vi "Main gScript UI.vi"() -> ()   [LabVIEW 2017]
uses:
  UI typedefs/gScript Controller Status.ctl
  gScript Interpreter/Type Definitions/Main Memory.ctl
  gScript Interpreter/Type Definitions/Memory Cell.ctl
  gScript Interpreter/Type Definitions/Memory Cell Type Enum.ctl
  gScript Interpreter/Type Definitions/Variable Table.ctl
  gScript Interpreter/Type Definitions/Variable.ctl
  Shared Components/Gantry Class/Type Definitions/Virtual Modes.ctl
  UI typedefs/gScript Controller Commands.ctl
  Shared Components/Gantry Class/Type Definitions/Init_Modes.ctl
  gScript Interpreter/gScript Interpreter.lvclass
  Application Utilities/Console Log/Console Log.lvclass
  Shared Components/Gantry Class/Gantry Class.lvclass
panel:
  out "Abort Async Request":bool=TRUE
  in  "Tab Control":enum32{"Control", "Memory"}(tab)
  in  "Execute":bool
  in  "Command Input":string
  in  "Virtual Mode":T1=enum."Virtual"
  out "Status":T2
  in  "Abort Script":bool
  in  "EXIT":bool
  in  "Config Root Directory":path
  in  "Pause Script":bool
  in  "Run Script":bool
  in  "Load Script":bool
  in  "Script Input":string
  in  "Save Script":bool
  out "Console":string
  in  "Variable Table":T3
  in  "Main Memory":T7
  in  "Memory Size":i32=16
  # "Documentation\nhttps://bit.ly/345jp8M"
  # "Command Input >"
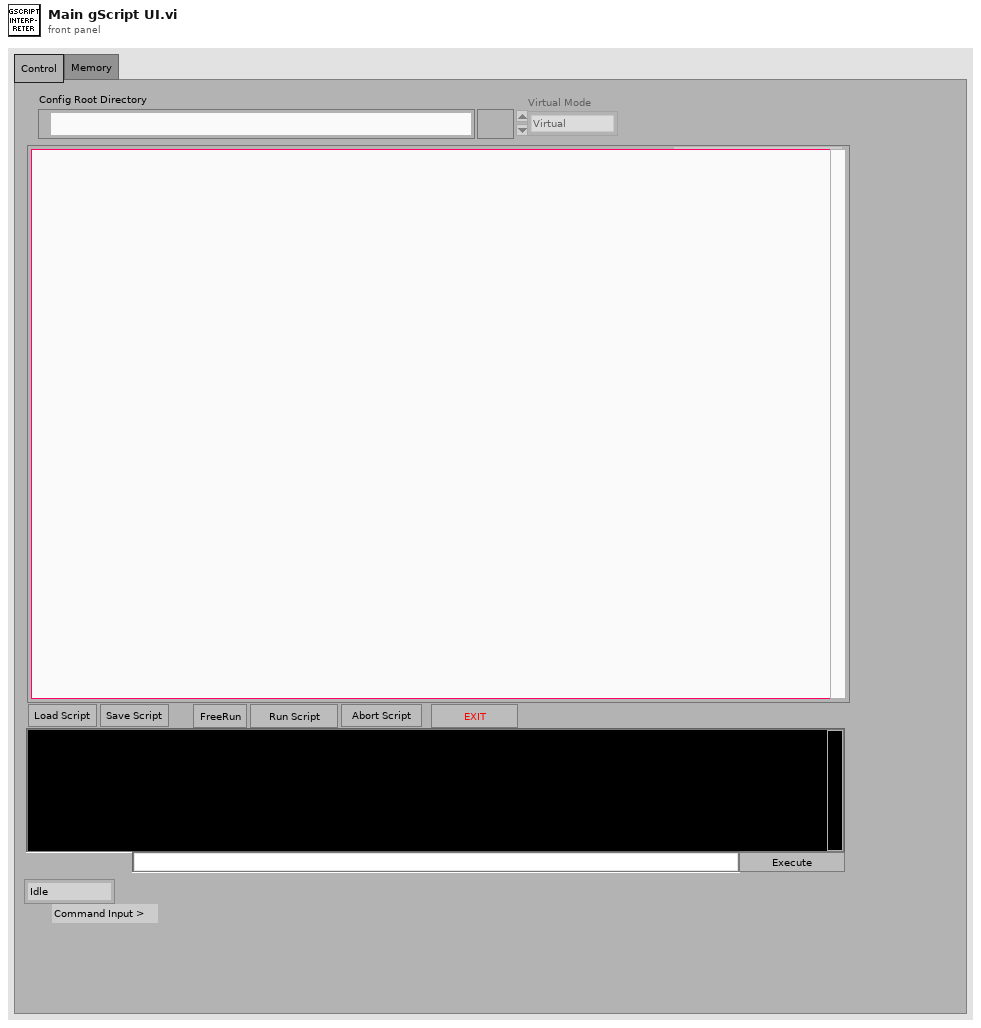
[diagram p1: front panel]
types:
  T1 = typedef "Virtual Modes.ctl" = enum16{"Nonvirtual", "Pseudovirtual", "Virtual"}
  T2 = typedef "gScript Controller Status.ctl" = enum16{"Idle", "Running", "Paused"}
  T3 = typedef "Variable Table.ctl" = T4[]
  T4 = typedef "Variable.ctl" = cluster{"Variable Name":string, "Memory Cell":T5}
  T5 = typedef "Memory Cell.ctl" = cluster{"type":T6, "x":dbl, "y":dbl, "z":dbl, "w":dbl}
  T6 = typedef "Memory Cell Type Enum.ctl" = enum16{"integer", "float", "vector", "rotation"}
  T7 = typedef "Main Memory.ctl" = T5[]
  T8 = enum8{"Enabled", "Disabled", "Disabled and Grayed Out"}
  T9 = typedef "gScript Controller Commands.ctl" = enum16{"Initialize", "Run Script", "Abort Script", "Exit", "Load Script", "Save Script", "Run Command"}
  T10 = cluster{"Variable Name":string, "Memory Cell":T5}[]
  T11 = typedef "Init_Modes.ctl" = enum16{"Full", "Robot Only", "Dispenser Only", "Cameras Only", "Robot and Cameras", "Robot and Cameras and Dispenser", "Manifold Only"}
  T12 = enum16{"open", "replace", "create", "open or create", "replace or create", "replace or create with confirmation"}
  T13 = cluster{"Shift":bool, "Ctrl":bool, "Alt":bool, "Cmd":bool, "Opt":bool}
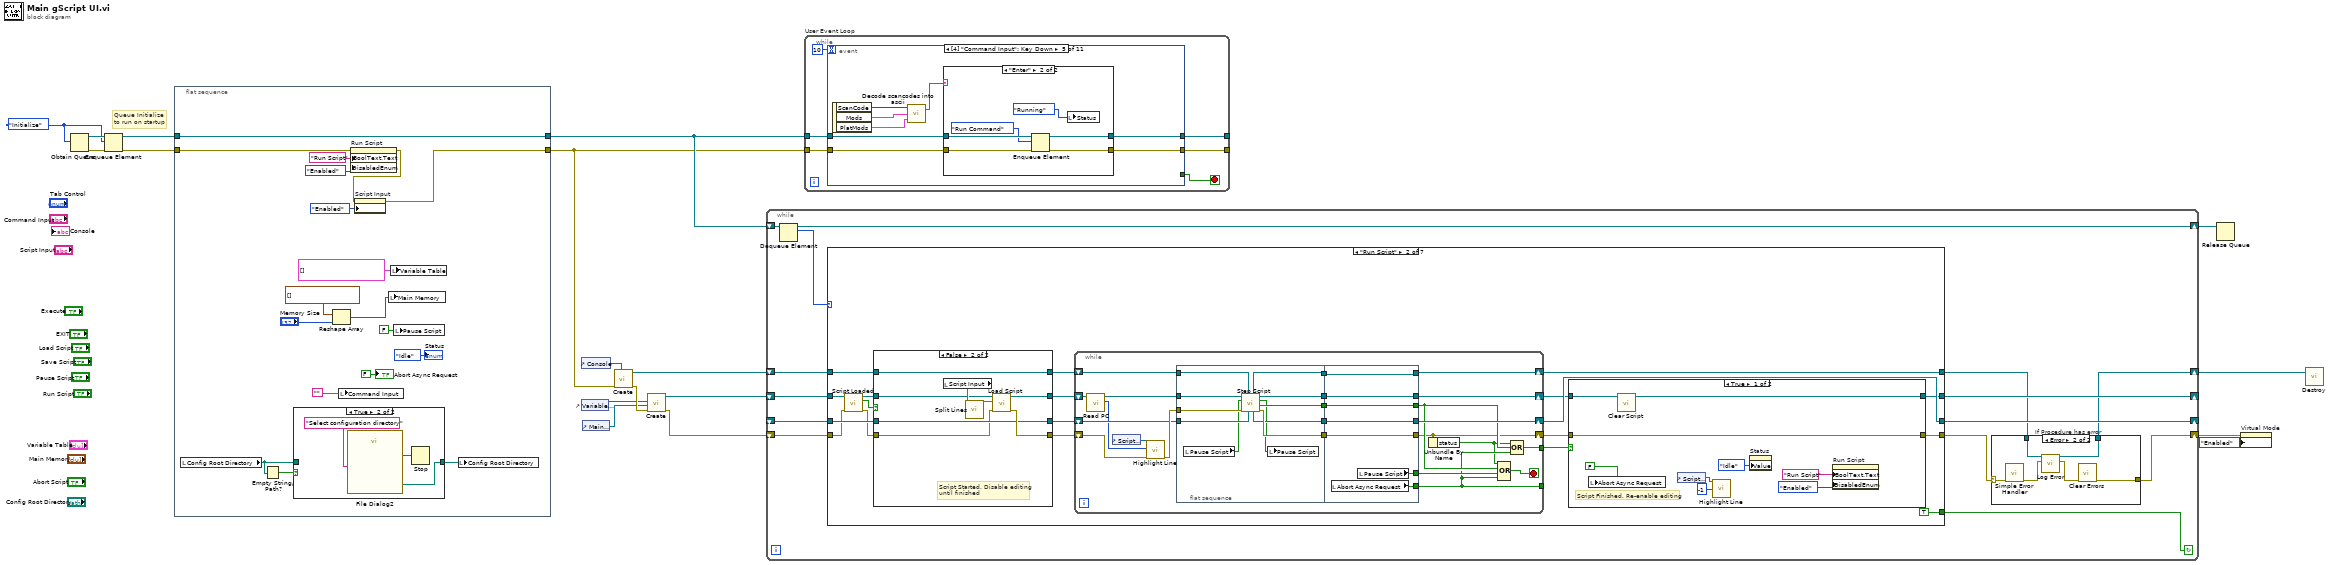
[diagram p0: block diagram]
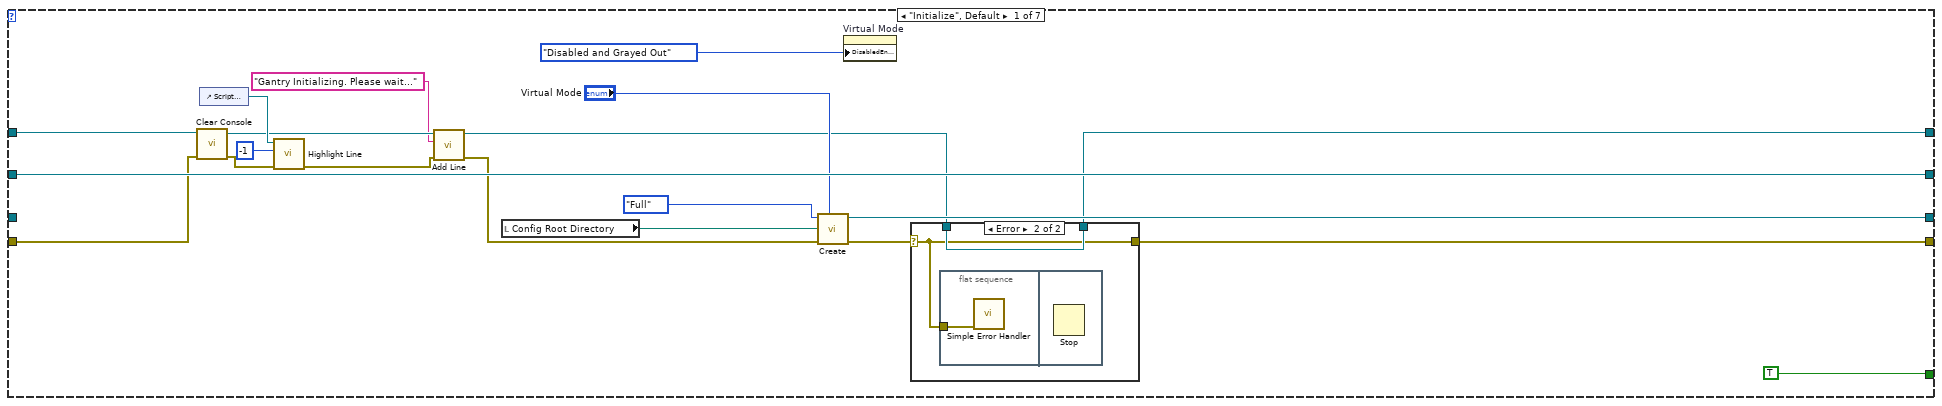
[diagram p4: hidden frame]
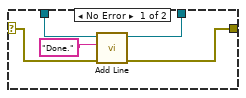
[diagram p5: hidden frame]
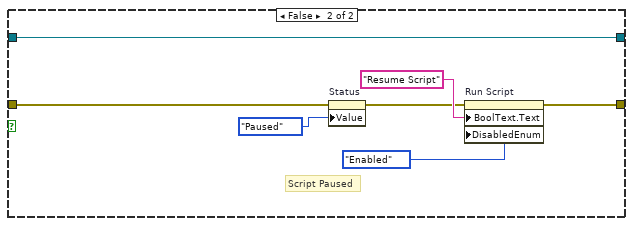
[diagram p7: hidden frame]
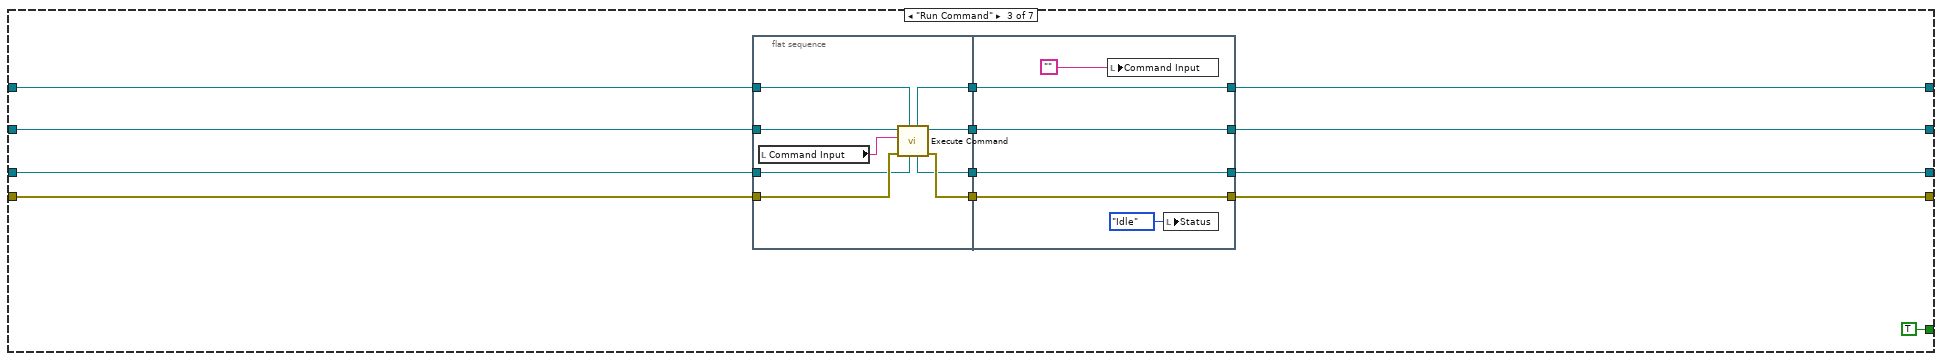
[diagram p8: hidden frame]
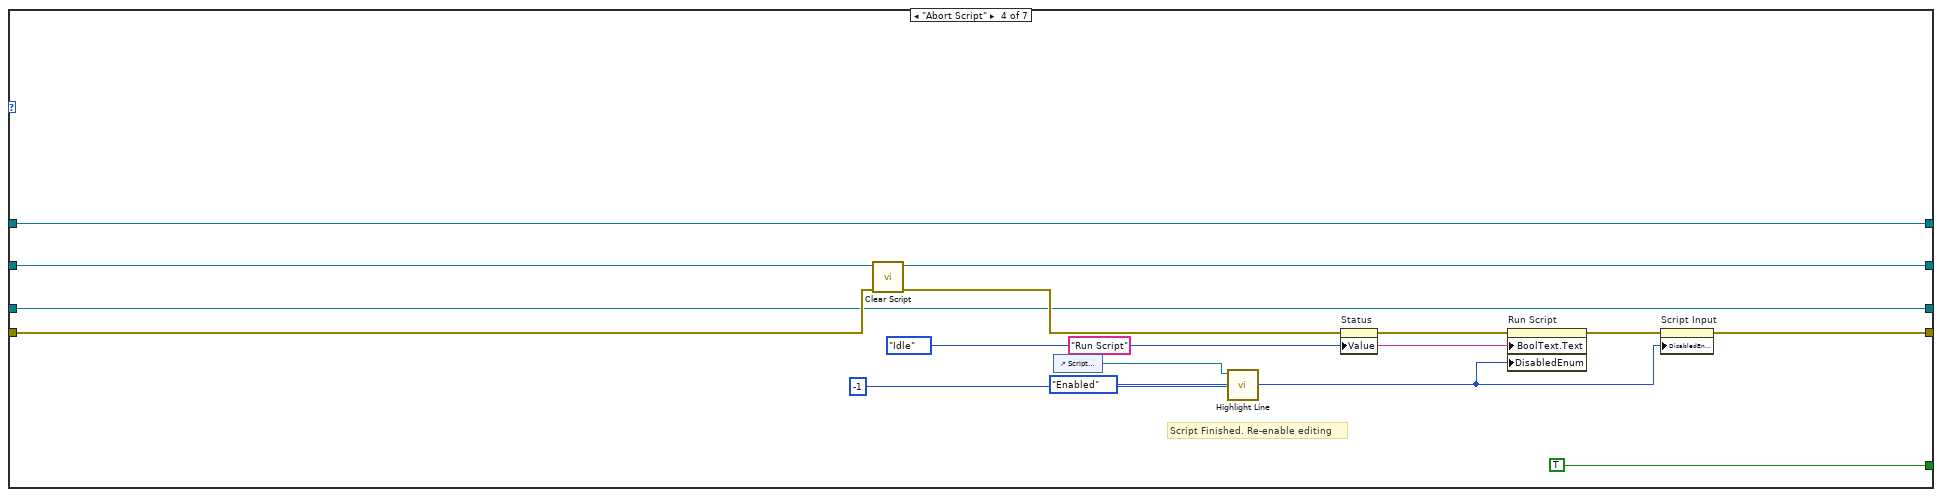
[diagram p9: hidden frame]
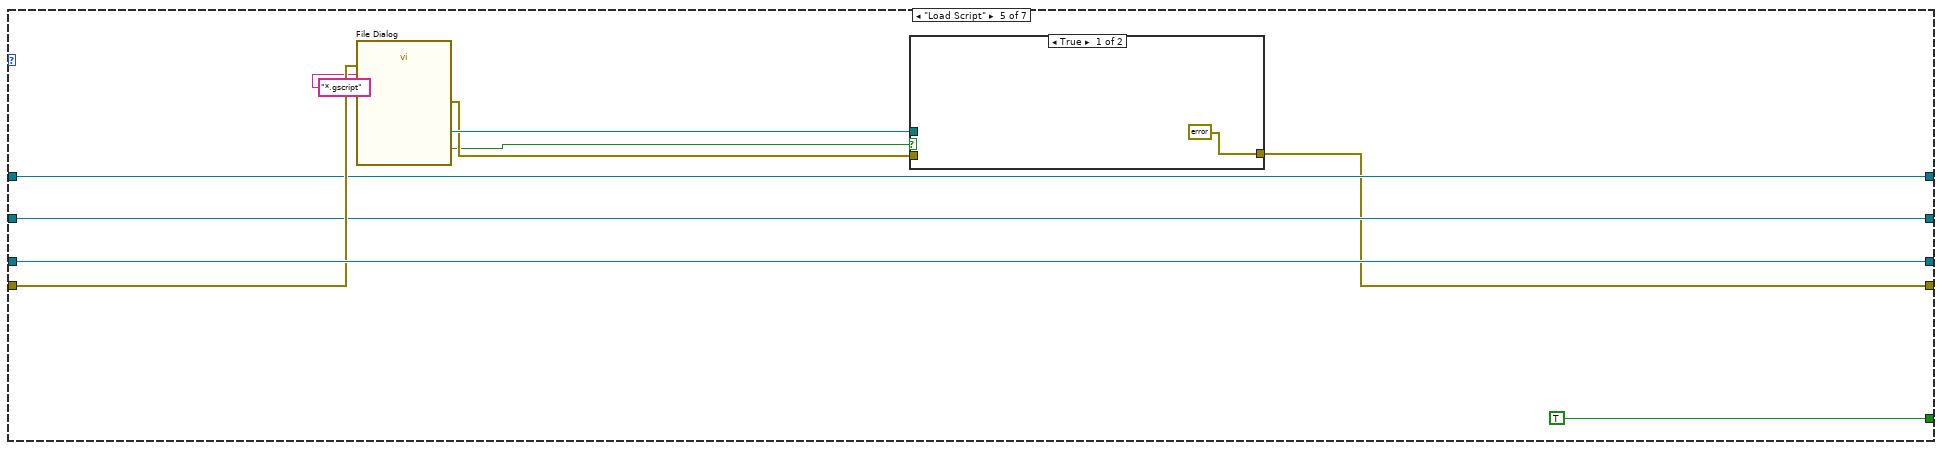
[diagram p10: hidden frame]
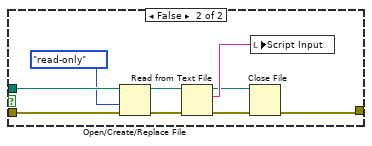
[diagram p11: hidden frame]
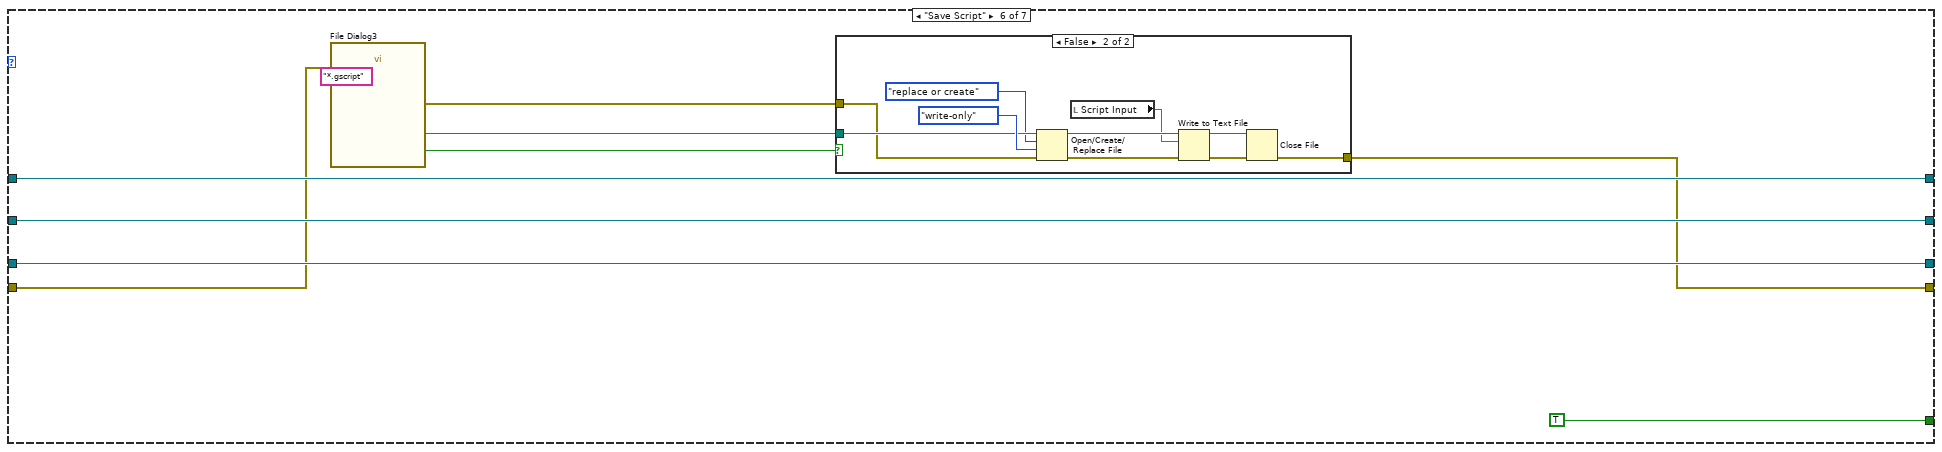
[diagram p12: hidden frame]
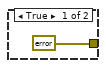
[diagram p13: hidden frame]
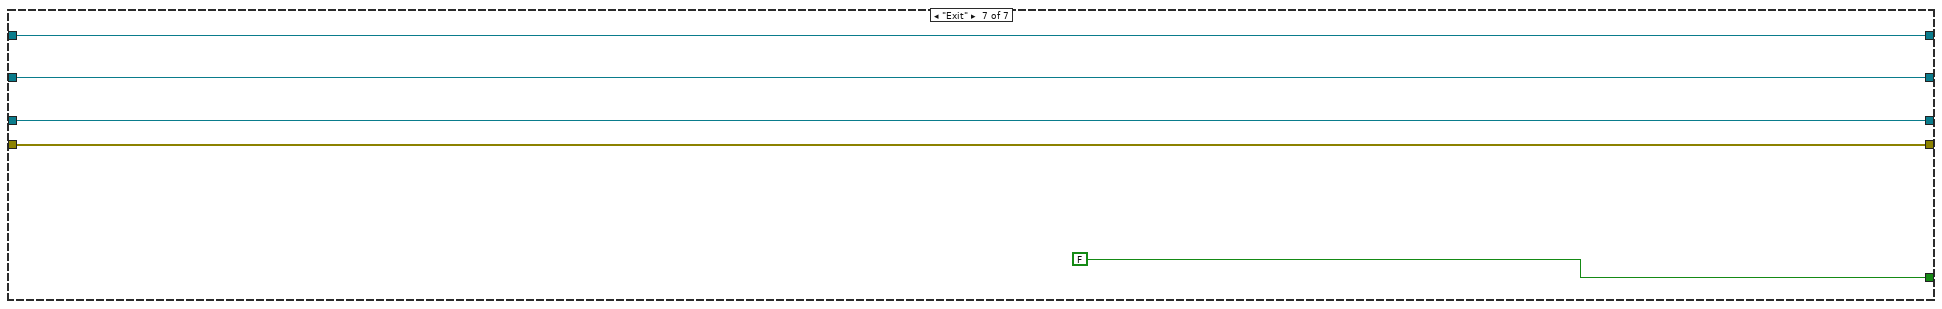
[diagram p14: hidden frame]
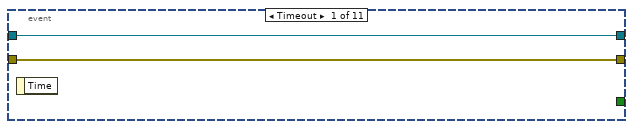
[diagram p15: hidden frame]
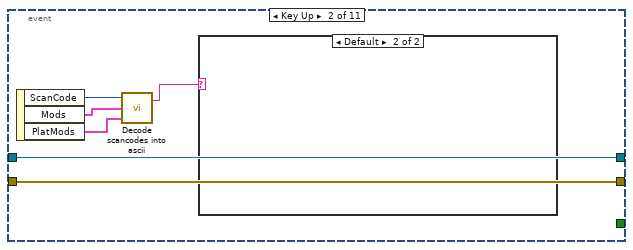
[diagram p16: hidden frame]
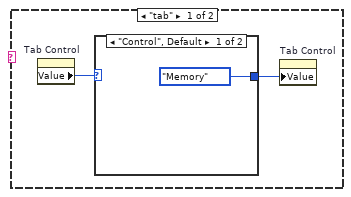
[diagram p17: hidden frame]
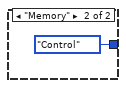
[diagram p18: hidden frame]
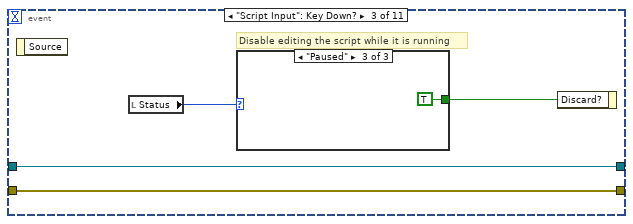
[diagram p19: hidden frame]
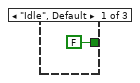
[diagram p20: hidden frame]
diagram:
  w15 = gScript_Controller_Commands."Initialize"
  # "Queue Initialize \nto run on startup"
  n1 = Obtain Queue(element data type=w15) -> (queue out=w17:refnum<queue>, error out=w16:errorcluster)  [unwired: 4 in, 1 out]
  n2 = Enqueue Element(queue=w17, element=w15, error in (no error)=w16) -> (queue out=w9:refnum<queue>, error out=w7:errorcluster)  [unwired: 1 in, 1 out]
  n3 = flat-sequence {
    tunnel: w9 -> [w36]
    tunnel: [w36] -> w8
    tunnel: w7 -> [w32]
    tunnel: [w29] -> w6
    frame #0 {
      n4 = local read "Config Root Directory"() -> (w22:path)
      n5 = Empty String/Path?(string/path=w22) -> (empty?=w21:bool)
      n6 = case shown="True" w21 {
        tunnel: w22 -> [w37 _]
        tunnel: [w37 w40] -> w20
        frame False {
        }
        frame True {
          n7 = call "File Dialog2"("prompt"="Select configuration directory") -> ("selected path"=w40:path, "cancelled"=w38:bool)  [unwired: 11 in, 2 out]
          n8 = Stop(stop? (T)=w38) -> ()
        }
      }
      n9 = Reshape Array(T5[] [] ("Main Memory"), "Memory Size") -> (w23:T5[])
      n10 = local write "Command Input"("") -> ()
      n11 = property on="Run Script" class="Bool (strict)"(error in=w32, "BoolText.Text"="Run Script" ("Boolean Text.Text"), "DisabledEnum"=T8."Enabled" ("Disabled")) -> (error out=w30:errorcluster)  [unwired: 1 in, 1 out]
      n12 = property on="Script Input" class="Str"(error in=w30, "DisabledEnum"=T8."Enabled" ("Disabled")) -> (error out=w29:errorcluster)  [unwired: 1 in, 1 out]
      n13 = local write "Main Memory"(w23) -> ()
      n14 = local write "Variable Table"(T10 [] ("Variable Table")) -> ()
      n15 = local write "Pause Script"(FALSE ("Pause Script")) -> ()
      n16 = local write "Config Root Directory"(w20) -> ()
      "Status" <- gScript_Controller_Status."Idle" ("Status")
      "Abort Async Request" <- FALSE ("Abort Requested")
    }
  }
  n17 = control-ref of="Variable Table"() -> (w4:refnum<vi>)
  n18 = control-ref of="Console"() -> (w18:refnum<vi>)
  n19 = control-ref of="Main Memory"() -> (w3:refnum<vi>)
  n20 = call "Create.vi"("Console"=w18, "error in"=w6) -> ("error out"=w11:errorcluster, "Console Log out"=w14:refnum<class "Console Log.lvclass">)  [unwired: 8 in]
  n21 = call "Create.vi"("error in (no error)"=w11, "Main Memory Ref"=w3, "Variable Table Ref"=w4) -> ("error out"=w10:errorcluster, "gScript Interpreter out"=w13:refnum<class "gScript Interpreter.lvclass">)  [unwired: 7 in]
  n22 = while {
    shift-right: [w41] -> w12
    shift-left: w14 -> [w52]
    shift-right: [w46] -> _
    shift-left: w13 -> [w51]
    shift-right: [w49] -> _
    shift-left: _ -> [w50]
    shift-right: [w43] -> w2
    shift-left: w10 -> [w48]
    shift-right: [w45] -> w5
    shift-left: w8 -> [w54]
    stop <- w47 continue-if-true
    n23 = Dequeue Element(queue=w54) -> (queue out=w45:refnum<queue>, element=w53:T9)  [unwired: 2 in, 2 out]
    n24 = case shown="\"Run Script\"" w53 {
      tunnel: w52 -> [w78 w100 w189 w211 w227 w249 w263]
      tunnel: w51 -> [w79 w98 w191 w214 w228 w250 w264]
      tunnel: w50 -> [_ w102 w185 w208 w231 w251 w265]
      tunnel: [w81 w93 w184 w208 w231 w251 w265] -> w49
      tunnel: w48 -> [w77 w96 w187 w213 w230 w246 w266]
      tunnel: [w66 w104 w186 w210 w223 w247 w266] -> w44
      tunnel: [TRUE TRUE TRUE TRUE TRUE TRUE FALSE] -> w47
      tunnel: [w67 w105 w188 w211 w227 w249 w263] -> w42
      tunnel: [w79 w91 w190 w212 w228 w250 w264] -> w46
      frame "Initialize", Default {
        n25 = call "Clear Console.vi"("error in (no error)"=w77, "Console Log in"=w78) -> ("error out"=w76:errorcluster, "Console Log out"=w72:refnum<class "Console Log.lvclass">)  [unwired: 8 in]
        n26 = control-ref of="Script Input"() -> (w75:refnum<vi>)
        n27 = call "Highlight Line.vi"("error in (no error)"=w76, "Line Number"=-1, "String Field In"=w75) -> ("error out"=w65:errorcluster)  [unwired: 7 in, 1 out]
        n28 = call "Add Line.vi"("error in"=w65, "String"="Gantry Initializing. Please wait...", "Console Log in"=w72) -> ("error out"=w69:errorcluster, "Console Log out"=w68:refnum<class "Console Log.lvclass">)  [unwired: 7 in]
        n29 = local read "Config Root Directory"() -> (w64:path)
        n30 = call "Create.vi"("Virtual Mode"="Virtual Mode", "error in"=w69, "Config Folder"=w64, "Init Mode"=Init_Modes."Full") -> ("error out"=w70:errorcluster, "Gantry out"=w81:refnum<class "Gantry Class.lvclass">)  [unwired: 6 in]
        n31 = property on="Virtual Mode" class="Enum (strict)"("DisabledEnum"=T8."Disabled and Grayed Out" ("Disabled")) -> ()  [unwired: 2 in, 2 out]
        n32 = case shown="Error" w70 {
          selector: w70 -> [w85 w88]
          tunnel: w68 -> [w87 w89]
          tunnel: [w86 w89] -> w67
          tunnel: [w84 w88] -> w66
          frame No Error {
            n33 = call "Add Line.vi"("error in"=w85, "String"="Done.", "Console Log in"=w87) -> ("error out"=w84:errorcluster, "Console Log out"=w86:refnum<class "Console Log.lvclass">)  [unwired: 7 in]
          }
          frame Error {
            n34 = flat-sequence {
              tunnel: w88 -> [w90]
              frame #0 {
                n35 = call <vilib>:"Simple Error Handler.vi"("error in (no error)"=w90) -> ()  [unwired: 4 in, 5 out]
              }
              frame #1 {
                n36 = Stop() -> ()  [unwired: 1 in]
              }
            }
          }
        }
      }
      frame "Run Script" {
        n37 = call-dynamic "Script Loaded.vi"("error in (no error)"=w96, "gScript Interpreter in"=w98) -> ("error out"=w95:errorcluster, "Script Loaded?"=w94:bool, "gScript Interpreter out"=w97:refnum<class "gScript Interpreter.lvclass">)  [unwired: 7 in]
        n38 = case shown="False" w94 {
          tunnel: w97 -> [w113 w120]
          tunnel: [w113 w119] -> w108
          tunnel: w95 -> [w110 w114]
          tunnel: [w110 w117] -> w107
          tunnel: w102 -> [w111 w116]
          tunnel: [w111 w116] -> w101
          tunnel: w100 -> [w112 w115]
          tunnel: [w112 w115] -> w99
          frame True {
          }
          frame False {
            # "Script Started. Disable editing\nuntil finished"
            n39 = local read "Script Input"() -> (w121:string)
            n40 = call "Split Lines.vi"("String In"=w121) -> ("Lines Out"=w118:string[])  [unwired: 10 in]
            n41 = call-dynamic "Load Script.vi"("error in (no error)"=w114, "Commands In"=w118, "gScript Interpreter in"=w120) -> ("error out"=w117:errorcluster, "gScript Interpreter out"=w119:refnum<class "gScript Interpreter.lvclass">)  [unwired: 7 in]
          }
        }
        n42 = while {
          shift-right: [w139] -> w106
          shift-left: w107 -> [w160]
          shift-right: [w157] -> w93
          shift-left: w101 -> [w158]
          shift-right: [w153] -> w92
          shift-left: w108 -> [w152]
          shift-right: [w154] -> w105
          shift-left: w99 -> [w155]
          tunnel: [w146] -> w103
          tunnel: [w145] -> _
          stop <- w148 stop-if-true
          n43 = call-dynamic "Read PC.vi"("gScript Interpreter in"=w152) -> ("PC"=w150:i32, "gScript Interpreter out"=w151:refnum<class "gScript Interpreter.lvclass">)  [unwired: 8 in, 1 out]
          n44 = control-ref of="Script Input"() -> (w156:refnum<vi>)
          n45 = call "Highlight Line.vi"("error in (no error)"=w160, "Line Number"=w150, "String Field In"=w156) -> ("error out"=w159:errorcluster)  [unwired: 7 in, 1 out]
          n46 = flat-sequence {
            tunnel: w159 -> [w171]
            tunnel: w158 -> [w169]
            tunnel: w155 -> [w167]
            tunnel: w151 -> [w164]
            tunnel: [w170] -> w144
            tunnel: [w168] -> w143
            tunnel: [w166] -> w142
            tunnel: [w165] -> w141
            tunnel: [w163] -> w140
            tunnel: [w173] -> w145
            tunnel: [w174] -> w147
            tunnel: [w172] -> w149
            tunnel: [w175] -> w153
            tunnel: [w176] -> w154
            tunnel: [w177] -> w157
            tunnel: [w178] -> w139
            tunnel: w144 -> [w178]
            tunnel: w143 -> [w177]
            tunnel: w142 -> [w176]
            tunnel: w141 -> [w175]
            tunnel: w140 -> [w174]
            frame #0 {
              n47 = local read "Pause Script"() -> (w162:bool)
              n48 = call-dynamic "Step Script.vi"("Gantry In"=w169, "Console Log In"=w167, "error in (no error)"=w171, "Pause in"=w162, "gScript Interpreter in"=w164) -> ("error out"=w170:errorcluster, "Finished"=w163:bool, "Pause out"=w161:bool, "gScript Interpreter out"=w165:refnum<class "gScript Interpreter.lvclass">, "Gantry Out"=w168:refnum<class "Gantry Class.lvclass">, "Console Log Out"=w166:refnum<class "Console Log.lvclass">)  [unwired: 1 in]
              n49 = local write "Pause Script"(w161) -> ()
            }
            frame #1 {
              n50 = local read "Abort Async Request"() -> (w173:bool)
              n51 = local read "Pause Script"() -> (w172:bool)
            }
          }
          n52 = Unbundle By Name(w139) -> ("status"=w138:bool)
          n53 = Compound Arithmetic op=OR(w138, w147, w149, w145) -> (w148:bool)
          n54 = Compound Arithmetic op=OR(w138, w147, w145) -> (w146:bool)
        }
        n55 = case shown="True" w103 {
          tunnel: w106 -> [w122 w137]
          tunnel: [w122 w132] -> w104
          tunnel: w92 -> [w125 w131]
          tunnel: [w124 w131] -> w91
          frame True {
            # "Script Finished. Re-enable editing"
            n56 = local write "Abort Async Request"(FALSE ("Abort Requested")) -> ()
            n57 = call-dynamic "Clear Script.vi"("gScript Interpreter in"=w125) -> ("gScript Interpreter out"=w124:refnum<class "gScript Interpreter.lvclass">)  [unwired: 9 in, 1 out]
            n58 = control-ref of="Script Input"() -> (w128:refnum<vi>)
            n59 = call "Highlight Line.vi"("Line Number"=-1, "String Field In"=w128) -> ()  [unwired: 8 in, 2 out]
            n60 = property on="Status" class="Enum (strict)"("Value"=gScript_Controller_Status."Idle" ("Status")) -> ()  [unwired: 2 in, 2 out]
            n61 = property on="Run Script" class="Bool (strict)"("BoolText.Text"="Run Script" ("Boolean Text.Text"), "DisabledEnum"=T8."Enabled" ("Disabled")) -> ()  [unwired: 2 in, 2 out]
          }
          frame False {
            # "Script Paused"
            n62 = property on="Status" class="Enum (strict)"(error in=w137, "Value"=gScript_Controller_Status."Paused" ("Status")) -> (error out=w133:errorcluster)  [unwired: 1 in, 1 out]
            n63 = property on="Run Script" class="Bool (strict)"(error in=w133, "BoolText.Text"="Resume Script" ("Boolean Text.Text"), "DisabledEnum"=T8."Enabled" ("Disabled")) -> (error out=w132:errorcluster)  [unwired: 1 in, 1 out]
          }
        }
      }
      frame "Run Command" {
        n64 = flat-sequence {
          tunnel: w191 -> [w200]
          tunnel: w189 -> [w198]
          tunnel: w187 -> [w196]
          tunnel: w185 -> [w194]
          tunnel: [w199] -> w182
          tunnel: [w197] -> w181
          tunnel: [w195] -> w180
          tunnel: [w193] -> w179
          tunnel: [w203] -> w184
          tunnel: [w204] -> w186
          tunnel: [w205] -> w188
          tunnel: [w206] -> w190
          tunnel: w182 -> [w206]
          tunnel: w181 -> [w205]
          tunnel: w180 -> [w204]
          tunnel: w179 -> [w203]
          frame #0 {
            n65 = local read "Command Input"() -> (w192:string)
            n66 = call-dynamic "Execute Command.vi"("Gantry In"=w194, "Console Log In"=w198, "error in (no error)"=w196, "Command"=w192, "gScript Interpreter in"=w200) -> ("error out"=w195:errorcluster, "gScript Interpreter out"=w199:refnum<class "gScript Interpreter.lvclass">, "Gantry Out"=w193:refnum<class "Gantry Class.lvclass">, "Console Log Out"=w197:refnum<class "Console Log.lvclass">)  [unwired: 2 in, 1 out]
          }
          frame #1 {
            n67 = local write "Command Input"("") -> ()
            n68 = local write "Status"(gScript_Controller_Status."Idle" ("Status")) -> ()
          }
        }
      }
      frame "Abort Script" {
        w216 = T8."Enabled" ("Disabled")
        # "Script Finished. Re-enable editing"
        n69 = call-dynamic "Clear Script.vi"("error in (no error)"=w213, "gScript Interpreter in"=w214) -> ("error out"=w215:errorcluster, "gScript Interpreter out"=w212:refnum<class "gScript Interpreter.lvclass">)  [unwired: 8 in]
        n70 = control-ref of="Script Input"() -> (w209:refnum<vi>)
        n71 = call "Highlight Line.vi"("Line Number"=-1, "String Field In"=w209) -> ()  [unwired: 8 in, 2 out]
        n72 = property on="Status" class="Enum (strict)"(error in=w215, "Value"=gScript_Controller_Status."Idle" ("Status")) -> (error out=w219:errorcluster)  [unwired: 1 in, 1 out]
        n73 = property on="Run Script" class="Bool (strict)"(error in=w219, "BoolText.Text"="Run Script" ("Boolean Text.Text"), "DisabledEnum"=w216) -> (error out=w217:errorcluster)  [unwired: 1 in, 1 out]
        n74 = property on="Script Input" class="Str"(error in=w217, "DisabledEnum"=w216) -> (error out=w210:errorcluster)  [unwired: 1 in, 1 out]
      }
      frame "Load Script" {
        n75 = call "File Dialog"("error in"=w230, "pattern (all files)"="*.gscript") -> ("selected path"=w225:path, "cancelled"=w222:bool, "error out"=w224:errorcluster)  [unwired: 10 in, 1 out]
        n76 = case shown="True" w222 {
          tunnel: w225 -> [_ w241]
          tunnel: w224 -> [_ w240]
          tunnel: [errorcluster {"status"=FALSE, "code"=0, "source"=""} ("error out") w233] -> w223
          frame True {
          }
          frame False {
            n77 = Open/Create/Replace File(file path (use dialog)=w241, error in=w240, access (0:read/write)=enum16{"read/write", "read-only", "write-only"}."read-only") -> (refnum out=w238:refnum<file>, error out=w237:errorcluster)  [unwired: 3 in, 1 out]
            n78 = Read from Text File(file (use dialog)=w238, error in=w237) -> (refnum out=w235:refnum<file>, text=w236:string, error out=w234:errorcluster)  [unwired: 2 in, 1 out]
            n79 = Close File(refnum=w235, error in=w234) -> (error out=w233:errorcluster)  [unwired: 1 out]
            n80 = local write "Script Input"(w236) -> ()
          }
        }
      }
      frame "Save Script" {
        n81 = call "File Dialog3"("error in"=w246, "pattern (all files)"="*.gscript") -> ("selected path"=w244:path, "cancelled"=w242:bool, "error out"=w243:errorcluster)  [unwired: 10 in, 1 out]
        n82 = case shown="False" w242 {
          tunnel: [errorcluster {"status"=FALSE, "code"=0, "source"=""} ("error out") w257] -> w247
          tunnel: w244 -> [_ w256]
          tunnel: w243 -> [_ w255]
          frame True {
          }
          frame False {
            n83 = Open/Create/Replace File(file path (use dialog)=w256, error in=w255, operation (0:open)=T12."replace or create", access (0:read/write)=enum16{"read/write", "read-only", "write-only"}."write-only") -> (refnum out=w261:refnum<file>, error out=w260:errorcluster)  [unwired: 2 in, 1 out]
            n84 = local read "Script Input"() -> (w254:string)
            n85 = Write to Text File(file (use dialog)=w261, text=w254, error in=w260) -> (refnum out=w259:refnum<file>, error out=w258:errorcluster)  [unwired: 1 in, 1 out]
            n86 = Close File(refnum=w259, error in=w258) -> (error out=w257:errorcluster)  [unwired: 1 out]
          }
        }
      }
      frame "Exit" {
      }
    }
    n87 = case "If Procedure has error" shown="Error" w44 {
      selector: w44 -> [w56 w62]
      tunnel: [w56 w61] -> w43
      tunnel: w42 -> [w55 w60]
      tunnel: [w55 w57] -> w41
      frame No Error {
      }
      frame Error {
        n88 = call <vilib>:"Simple Error Handler.vi"("error in (no error)"=w62) -> ("error out"=w59:errorcluster)  [unwired: 4 in, 4 out]
        n89 = call "Log Error.vi"("error in"=w59, "Console Log in"=w60) -> ("error out"=w58:errorcluster, "Console Log out"=w57:refnum<class "Console Log.lvclass">)  [unwired: 8 in]
        n90 = call <vilib>:"Clear Errors.vi"("error in (no error)"=w58) -> ("error out"=w61:errorcluster)  [unwired: 5 in, 1 out]
      }
    }
  }
  n91 = while "User Event Loop" {
    tunnel: w8 -> [w268]
    tunnel: [w271] -> _
    tunnel: w6 -> [w270]
    tunnel: [w269] -> _
    stop <- w272 stop-if-true
    n92 = event shown="[4] \"Command Input\": Key Down" {
      selector: _ -> [_ _ _ _ _ _ _ _ _ _ _]
      dyn-events: _ -> [_ _ _ _ _ _ _ _ _ _ _]
      timeout: 10 -> [_ _ _ _ _ _ _ _ _ _ _]
      tunnel: [_ _ _ _ _ _ _ _ _ TRUE ("T button?") w394] -> w272
      tunnel: w268 -> [w275 w281 w289 w297 w313 w326 w348 w364 w377 w391 w393]
      tunnel: [w275 w281 w289 w295 w311 w323 w347 w361 w375 w390 w393] -> w271
      tunnel: w270 -> [w274 w280 w288 w296 w312 w325 w346 w363 w376 w389 w392]
      tunnel: [w274 w280 w288 w294 w310 w324 w345 w360 w374 w388 w392] -> w269
      event Timeout {
        n93 = event-data() -> ()  [unwired: 1 in, 1 out]
      }
      event Key Up {
        n94 = event-data() -> ("ScanCode"=w279:i16, "Mods"=w278:cluster{"Num Pad":bool, "Menu Key":bool}, "PlatMods"=w277:T13)  [unwired: 1 in]
        n95 = call "Decode scancodes into ascii.vi"("PlatMods"=w277, "Mods"=w278, "ScanCode"=w279) -> ("String"=w276:string)  [unwired: 1 out]
        n96 = case shown="Default" w276 {
          frame "tab" {
            n97 = property on="Tab Control" class="TabCtl (strict)"() -> ("Value"=w283:enum32{"Control", "Memory"})  [unwired: 2 in, 2 out]
            n98 = case shown="\"Control\", Default" w283 {
              tunnel: [enum32{"Control", "Memory"}."Memory" ("Tab Control") enum32{"Control", "Memory"}."Control" ("Tab Control")] -> w282
              frame "Control", Default {
              }
              frame "Memory" {
              }
            }
            n99 = property on="Tab Control" class="TabCtl (strict)"("Value"=w282) -> ()  [unwired: 2 in, 2 out]
          }
          frame Default {
          }
        }
      }
      event "Script Input": Key Down? {
        # "Disable editing the script while it is running"
        n100 = event-data() -> ()  [unwired: 1 in, 1 out]
        n101 = local read "Status"() -> (w287:T2)
        n102 = case shown="\"Paused\"" w287 {
          tunnel: [FALSE TRUE TRUE] -> w286
          frame "Idle", Default {
          }
          frame "Running" {
          }
          frame "Paused" {
          }
        }
        n103 = event-data("Discard?"=w286) -> ()  [unwired: 1 in, 1 out]
      }
      event "Execute": Value Change {
        n104 = event-data() -> ("NewVal"=w293:bool)  [unwired: 1 in]
        n105 = case shown="True" w293 {
          tunnel: w297 -> [w298 w305]
          tunnel: w296 -> [w299 w302]
          tunnel: [w298 w304] -> w295
          tunnel: [w299 w301] -> w294
          frame False {
          }
          frame True {
            n106 = Enqueue Element(queue=w305, element=gScript_Controller_Commands."Run Command", error in (no error)=w302) -> (queue out=w304:refnum<queue>, error out=w301:errorcluster)  [unwired: 1 in, 1 out]
            n107 = local write "Status"(gScript_Controller_Status."Running" ("Status")) -> ()
          }
        }
      }
      event "Command Input": Key Down {
        n108 = event-data() -> ("ScanCode"=w309:i16, "Mods"=w308:cluster{"Num Pad":bool, "Menu Key":bool}, "PlatMods"=w307:T13)  [unwired: 1 in]
        n109 = call "Decode scancodes into ascii.vi"("PlatMods"=w307, "Mods"=w308, "ScanCode"=w309) -> ("String"=w306:string)  [unwired: 1 out]
        n110 = case shown="\"Enter\"" w306 {
          tunnel: w313 -> [w314 w321]
          tunnel: w312 -> [w315 w318]
          tunnel: [w314 w320] -> w311
          tunnel: [w315 w317] -> w310
          frame Default {
          }
          frame "Enter" {
            n111 = Enqueue Element(queue=w321, element=gScript_Controller_Commands."Run Command", error in (no error)=w318) -> (queue out=w320:refnum<queue>, error out=w317:errorcluster)  [unwired: 1 in, 1 out]
            n112 = local write "Status"(gScript_Controller_Status."Running" ("Status")) -> ()
          }
        }
      }
      event "Run Script": Mouse Up {
        n113 = event-data() -> ()  [unwired: 1 in, 1 out]
        n114 = local read "Status"() -> (w322:T2)
        n115 = case shown="\"Idle\"" w322 {
          tunnel: w326 -> [w328 w336 w343]
          tunnel: w325 -> [w327 w335 w342]
          tunnel: [w327 w334 w339] -> w324
          tunnel: [w328 w333 w340] -> w323
          frame "Running" {
          }
          frame "Idle" {
            n116 = Enqueue Element(queue=w336, element=gScript_Controller_Commands."Run Script", error in (no error)=w335) -> (queue out=w333:refnum<queue>, error out=w334:errorcluster)  [unwired: 1 in, 1 out]
            n117 = property on="Run Script" class="Bool (strict)"("BoolText.Text"="Running" ("Boolean Text.Text"), "DisabledEnum"=T8."Disabled and Grayed Out" ("Disabled")) -> ()  [unwired: 2 in, 2 out]
            n118 = local write "Status"(gScript_Controller_Status."Running" ("Status")) -> ()
          }
          frame "Paused" {
            n119 = Enqueue Element(queue=w343, element=gScript_Controller_Commands."Run Script", error in (no error)=w342) -> (queue out=w340:refnum<queue>, error out=w339:errorcluster)  [unwired: 1 in, 1 out]
            n120 = property on="Run Script" class="Bool (strict)"("BoolText.Text"="Running" ("Boolean Text.Text"), "DisabledEnum"=T8."Disabled and Grayed Out" ("Disabled")) -> ()  [unwired: 2 in, 2 out]
            n121 = local write "Status"(gScript_Controller_Status."Running" ("Status")) -> ()
          }
        }
      }
      event "Abort Script": Mouse Up {
        n122 = event-data() -> ()  [unwired: 1 in, 1 out]
        n123 = local read "Status"() -> (w349:T2)
        n124 = case shown="\"Running\"" w349 {
          tunnel: w348 -> [w351 w353 w358]
          tunnel: [w351 w353 w357] -> w347
          tunnel: w346 -> [w350 w352 w356]
          tunnel: [w350 w352 w355] -> w345
          frame "Idle", Default {
          }
          frame "Running" {
            n125 = local write "Abort Async Request"(TRUE ("Abort Requested")) -> ()
          }
          frame "Paused" {
            n126 = Enqueue Element(queue=w358, element=gScript_Controller_Commands."Abort Script", error in (no error)=w356) -> (queue out=w357:refnum<queue>, error out=w355:errorcluster)  [unwired: 1 in, 1 out]
          }
        }
      }
      event "Load Script": Mouse Up {
        n127 = event-data() -> ()  [unwired: 1 in, 1 out]
        n128 = local read "Status"() -> (w362:T2)
        n129 = case shown="\"Idle\", Default" w362 {
          tunnel: w364 -> [w369 w372]
          tunnel: w363 -> [w368 w371]
          tunnel: [w366 w372] -> w361
          tunnel: [w367 w371] -> w360
          frame "Idle", Default {
            n130 = Enqueue Element(queue=w369, element=gScript_Controller_Commands."Load Script", error in (no error)=w368) -> (queue out=w366:refnum<queue>, error out=w367:errorcluster)  [unwired: 1 in, 1 out]
          }
          frame "Running", "Paused" {
            n131 = One Button Dialog(message="Cannot Load while Script is Running or Paused\nAbort or finish running script first.") -> ()  [unwired: 1 in, 1 out]
          }
        }
      }
      event "Save Script": Mouse Up {
        n132 = event-data() -> ()  [unwired: 1 in, 1 out]
        n133 = local read "Status"() -> (w373:T2)
        n134 = case shown="\"Idle\", Default" w373 {
          tunnel: w377 -> [w382 w385]
          tunnel: w376 -> [w381 w384]
          tunnel: [w379 w385] -> w375
          tunnel: [w380 w384] -> w374
          frame "Idle", Default {
            n135 = Enqueue Element(queue=w382, element=gScript_Controller_Commands."Save Script", error in (no error)=w381) -> (queue out=w379:refnum<queue>, error out=w380:errorcluster)  [unwired: 1 in, 1 out]
          }
          frame "Running", "Paused" {
            n136 = One Button Dialog(message="Cannot Save while Script is Running or Paused\nAbort or finish running script first.") -> ()  [unwired: 1 in, 1 out]
          }
        }
      }
      event "EXIT": Mouse Up {
        n137 = event-data() -> ()  [unwired: 1 in, 1 out]
        n138 = Enqueue Element(queue=w391, element=gScript_Controller_Commands."Exit", error in (no error)=w389) -> (queue out=w390:refnum<queue>, error out=w388:errorcluster)  [unwired: 1 in, 1 out]
      }
      event Panel Close? {
        n139 = event-data() -> ()  [unwired: 1 in, 1 out]
        n140 = Two Button Dialog(message="Are you sure you want to quit?", 1:"Return" ("F button name (\"Cancel\")"), 2:"Quit" ("T button name (\"OK\")")) -> (T button?=w394:bool)
        n141 = event-data("Discard?"=TRUE) -> ()  [unwired: 1 in, 1 out]
      }
    }
  }
  n142 = Release Queue(queue=w5) -> ()  [unwired: 2 in, 3 out]
  n143 = property on="Virtual Mode" class="Enum (strict)"(error in=w2, "DisabledEnum"=T8."Enabled" ("Disabled")) -> ()  [unwired: 1 in, 2 out]
  n144 = call "Destroy.vi"("Console Log in"=w12) -> ()  [unwired: 10 in, 1 out]
